vi "Close.vi"(8 "error in (no error)":errorcluster, 11 "Filter Wheel in":refnum<class "Filter Wheel.lvclass">) -> (0 "error out":errorcluster, 3 "Filter Wheel out":refnum<class "Filter Wheel.lvclass">)   [LabVIEW 2021, in "Filter Wheel.lvclass"]
uses:
  Filter Wheel.lvclass
  Filter Wheel.lvclass/Filter Wheel.ctl
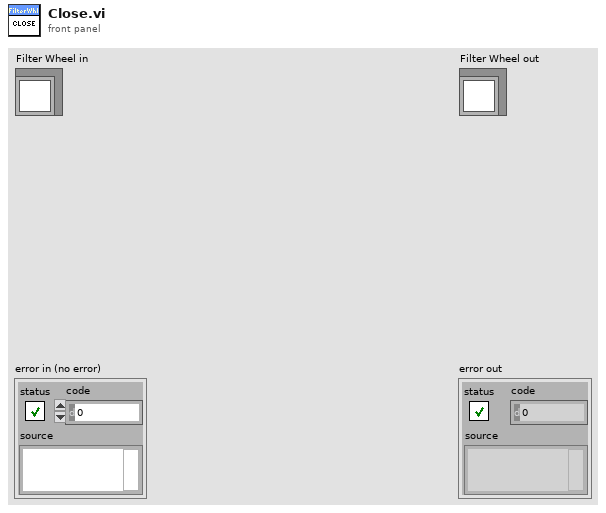
[diagram p1: front panel]
types:
  T1 = typedef "Filter Wheel.lvclass/Filter Wheel configuration.ctl" = cluster{"Num Wheels":i32, "Filters":T2[], "Invalid Combinations":i32[][], "Addr":refnum<visa-resource-name>, "Name":string, "Simulate":bool, "Homing Parameters":T3, "Default Speed":u16}
  T2 = typedef "Filter Wheel.lvclass/Filter Wheel Details.ctl" = cluster{"Names":string[], "Relative Position":i32[], "Wheel Name":string}
  T3 = typedef "Filter Wheel Arduino Homing cluster.ctl" = cluster{"Direction (F: CW)":bool, "Speed":i32, "Accel":i32, "Min Distance":i32, "Short Leg":i32, "Error Cnts":i32}
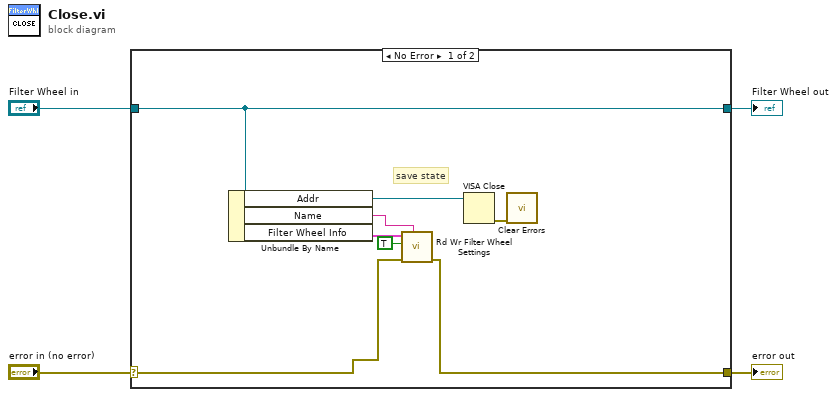
[diagram p0: block diagram]
diagram:
  n1 = case shown="No Error" "error in (no error)" {
    selector: "error in (no error)" -> [w9 w14]
    tunnel: [w8 w14] -> w3
    tunnel: [w12 w13] -> w1
    tunnel: "Filter Wheel in" -> [w12 w13]
    frame No Error {
      # "save state"
      n2 = Unbundle By Name(w12) -> ("Addr"=w6:refnum<visa-resource-name>, "Name"=w7:string, "Filter Wheel Info"=w11:T1)
      n3 = call "Rd Wr Filter Wheel Settings.vi"("Wheel Name"=w7, "error in (no error)"=w9, "Write? (F:Read)"=TRUE, "Filter Wheel Settings"=w11) -> ("error out"=w8:errorcluster)  [unwired: 6 in, 1 out]
      n4 = VISA Close(VISA resource name=w6) -> (error out=w5:errorcluster)  [unwired: 1 in]
      n5 = call <vilib>:"Clear Errors.vi"("error in (no error)"=w5) -> ()  [unwired: 5 in, 2 out]
    }
    frame Error {
    }
  }
  "error out" <- w3
  "Filter Wheel out" <- w1
